vi "Increment File Name.vi"(6 "Movie auto-numbering":T1=enum."Movie series", 9 "Fields":i32, 10 "Movie Index":i32, 11 "Input Path":path) -> (3 "Output Path":path)   [LabVIEW 2023]
uses:
  Type Defs/Movie auto-numbering.ctl
  <vilib>/regexp/Match Regular Expression.xnode
panel:
  out "Files":path[](array[path])
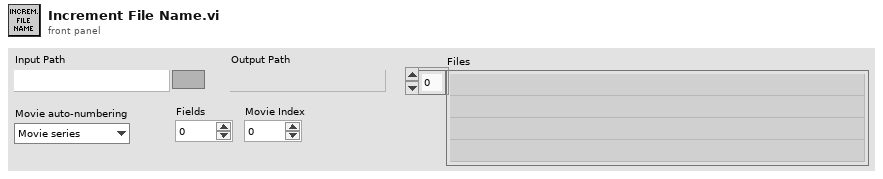
[diagram p1: front panel]
types:
  T1 = typedef "Movie auto-numbering.ctl" = enum16{"Single movie", "Movie series", "Multi-lane series"}
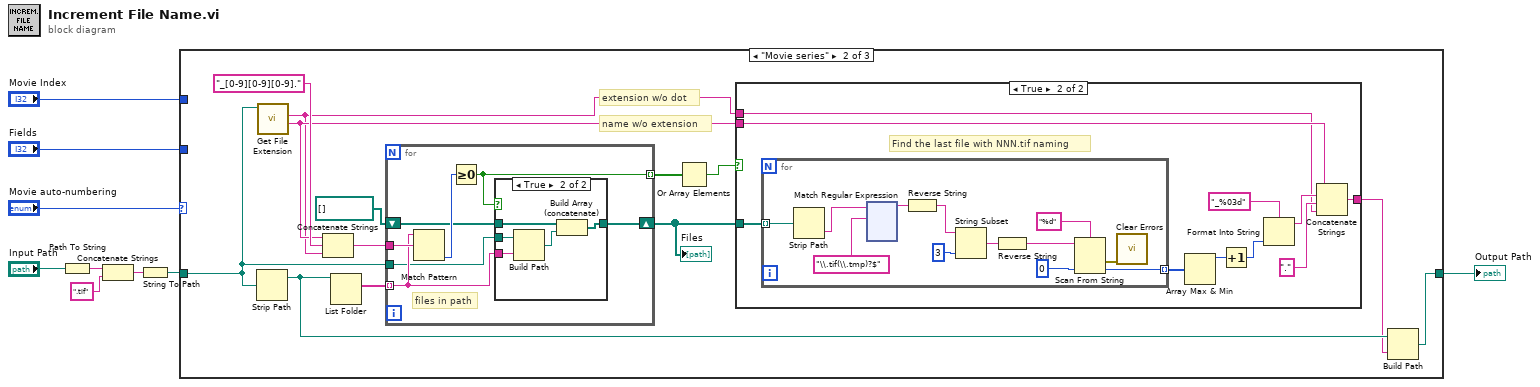
[diagram p0: block diagram]
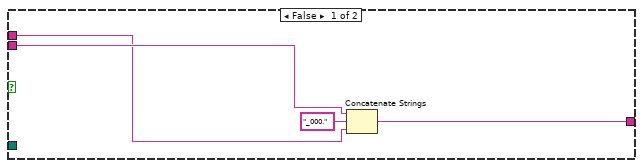
[diagram p3: hidden frame]
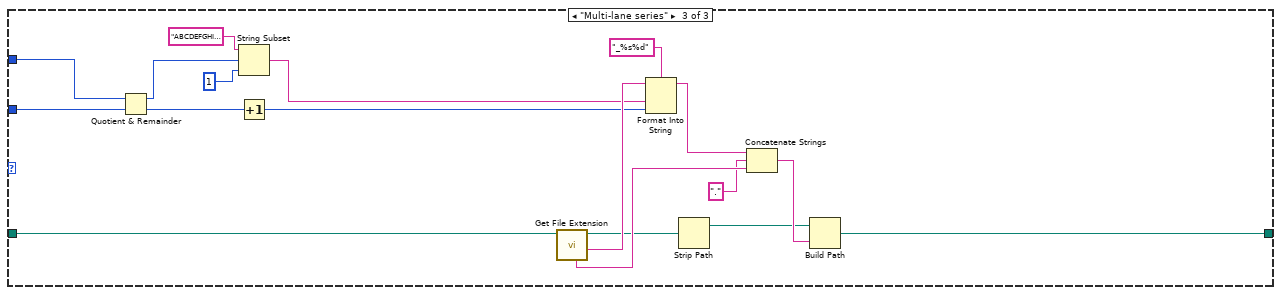
[diagram p5: hidden frame]
diagram:
  n1 = Path To String(path="Input Path") -> (string=w7:string)
  n2 = Concatenate Strings(w7, ".tif" ("string")) -> (w8:string)
  n3 = String To Path(string=w8) -> (path=w4:path)
  n4 = case shown="\"Movie series\"" "Movie auto-numbering" {
    tunnel: [w10 w13 w189] -> w9
    tunnel: w4 -> [w10 w11 w195]
    tunnel: "Movie Index" -> [_ _ w197]
    tunnel: "Fields" -> [_ _ w196]
    frame "Single movie", Default {
    }
    frame "Movie series" {
      # "extension w/o dot"
      # "name w/o extension"
      n5 = Strip Path(path=w11) -> (stripped path=w15:path)  [unwired: 1 out]
      n6 = call <vilib>:"Get File Extension.vi"("file"=w11) -> ("filename without extension"=w18:string, "lowercase file extension"=w17:string)  [unwired: 6 in, 3 out]
      n7 = Concatenate Strings(w18, "_[0-9][0-9][0-9]." ("string"), w17) -> (w21:string)
      n8 = List Folder(path=w15) -> (filenames=w23:string[])  [unwired: 3 in, 3 out]
      n9 = for {
        tunnel: w23 -> [w168] mode=indexing
        tunnel: w21 -> [w173]
        tunnel: [w171] -> w20 mode=indexing
        shift-right: [w170] -> w16
        shift-left: path[] [] -> [w169]
        tunnel: w11 -> [w167]
        # "files in path"
        n10 = Match Pattern(string=w168, regular expression=w173) -> (offset past match=w172:i32)  [unwired: 1 in, 3 out]
        n11 = Greater Or Equal To 0?(x=w172) -> (x >= 0?=w171:bool)
        n12 = case shown="True" w171 {
          tunnel: w168 -> [_ w176]
          tunnel: [w174 w179] -> w170
          tunnel: w169 -> [w174 w178]
          tunnel: w167 -> [_ w177]
          frame False {
          }
          frame True {
            n13 = Build Path(base path=w177, name or relative path=w176) -> (appended path=w175:path)
            n14 = Build Array (concatenate)(w178, w175) -> (w179:path[])
          }
        }
      }
      "Files" <- w16
      n15 = Or Array Elements(Boolean array=w20) -> (logical OR=w19:bool)
      n16 = case shown="True" w19 {
        tunnel: w18 -> [w26 w31]
        tunnel: w17 -> [w25 w29]
        tunnel: w16 -> [_ w37]
        tunnel: [w24 w32] -> w14
        frame False {
          n17 = Concatenate Strings(w26, "_000." ("string"), w25) -> (w24:string)
        }
        frame True {
          # "Find the last file with NNN.tif naming"
          n18 = for {
            tunnel: w37 -> [w41] mode=indexing
            tunnel: [w47] -> w28 mode=indexing
            n19 = Strip Path(path=w41) -> (name=w39:string)  [unwired: 1 out]
            n20 = xnode "Match Regular Expression"("input string"=w39, "regular expression"="\\.tif(\\.tmp)?$") -> ("before match"=w40:string)  [unwired: 4 in, 4 out]
            n21 = Reverse String(1:w40) -> (0:w45:string)
            n22 = String Subset(string=w45, length (rest)=3 ("length (rest)")) -> (substring=w44:string)  [unwired: 1 in]
            n23 = Reverse String(1:w44) -> (0:w43:string)
            n24 = Scan From String(format string="%d", input string=w43, default 1=0 ("default value 1")) -> (error out=w46:errorcluster, output 1=w47:i32)  [unwired: 2 in, 2 out]
            n25 = call <vilib>:"Clear Errors.vi"("error in (no error)"=w46) -> ()  [unwired: 5 in, 2 out]
          }
          n26 = Array Max & Min(array=w28) -> (max value=w34:i32)  [unwired: 3 out]
          n27 = Increment(x=w34) -> (x+1=w33:i32)
          n28 = Format Into String(format string="_%03d", w33) -> (resulting string=w36:string)  [unwired: 2 in, 1 out]
          n29 = Concatenate Strings(w31, w36, "." ("string"), w29) -> (w32:string)
        }
      }
      n30 = Build Path(base path=w15, name or relative path=w14) -> (appended path=w13:path)
    }
    frame "Multi-lane series" {
      n31 = Quotient & Remainder(x=w197, y=w196) -> (x-y*floor(x/y)=w183:i32, floor(x/y)=w181:i32)
      n32 = String Subset(string="ABCDEFGHIJKLMNOPQRSTUVWXYZ", offset (0)=w183, length (rest)=1 ("length (rest)")) -> (substring=w182:string)
      n33 = Increment(x=w181) -> (x+1=w180:i32)
      n34 = call <vilib>:"Get File Extension.vi"("file"=w195) -> ("filename without extension"=w194:string, "dup file"=w187:path, "unmodified file extension"=w191:string)  [unwired: 6 in, 2 out]
      n35 = Format Into String(format string="_%s%d", initial string=w194, w182, w180) -> (resulting string=w192:string)  [unwired: 1 in, 1 out]
      n36 = Strip Path(path=w187) -> (stripped path=w186:path)  [unwired: 1 out]
      n37 = Concatenate Strings(w192, "." ("string"), w191) -> (w188:string)
      n38 = Build Path(base path=w186, name or relative path=w188) -> (appended path=w189:path)
    }
  }
  "Output Path" <- w9
